vi "未命名 5.vi"() -> ()   [LabVIEW 2017]
panel:
  in  "停止按钮":bool
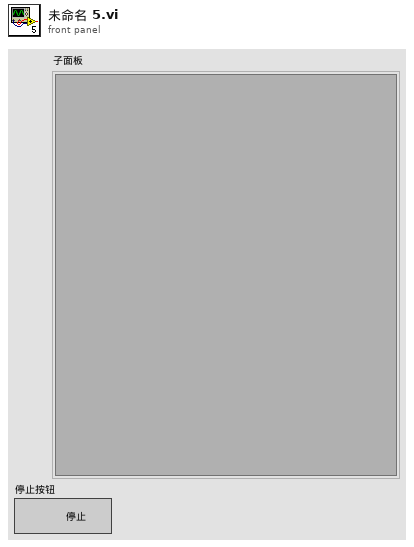
[diagram p1: front panel]
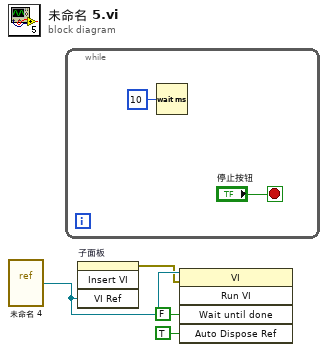
[diagram p0: block diagram]
diagram:
  n1 = vi-ref "未命名 4.vi"() -> (w4:refnum<vi>)
  n2 = while {
    stop <- "停止按钮" stop-if-true
    n3 = Wait (ms)(milliseconds to wait=u32 10 ("等待时间（毫秒）")) -> ()  [unwired: 1 out]
  }
  n4 = invoke on="子面板" class="SubPnl" method="Insert VI"("VI Ref"=w4) -> (error out=w3:errorcluster)  [unwired: 3 in, 3 out]
  n5 = invoke class="VI" method="Run VI"(reference=w4, error in=w3, "Wait until done"=FALSE ("结束前等待"), "Auto Dispose Ref"=TRUE ("自动销毁引用")) -> ()  [unwired: 1 in, 5 out]
